vi "Event Structure Details.vi"() -> ()   [LabVIEW 2023]
panel:
  in  "State mashine Time out control":i32
  out "Numeric":i32
  in  "stop":bool
  in  "OK Button":bool
  out "time string":string
  out "Waveform Chart":dbl(graph)
  # "Виж разликата когато е -1 и > -1"
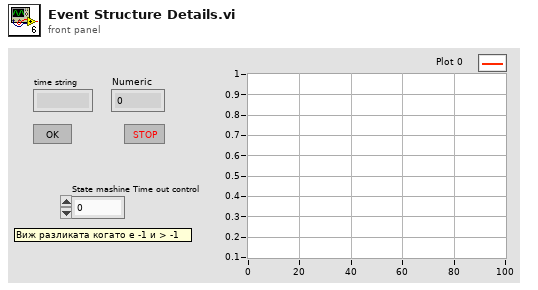
[diagram p1: front panel]
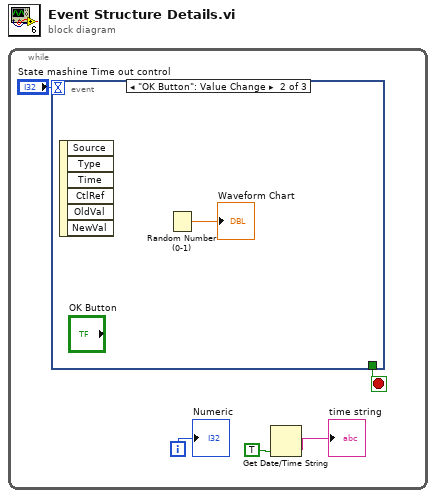
[diagram p0: block diagram]
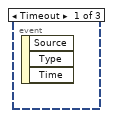
[diagram p2: hidden frame]
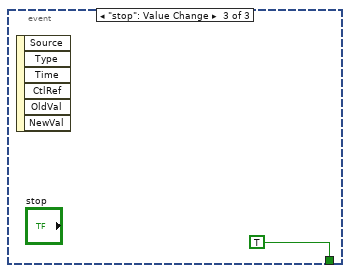
[diagram p3: hidden frame]
diagram:
  n1 = while {
    i -> [w3]
    stop <- w4 stop-if-true
    n2 = event shown="[1] \"OK Button\": Value Change" {
      selector: _ -> [_ _ _]
      dyn-events: _ -> [_ _ _]
      timeout: "State mashine Time out control" -> [_ _ _]
      tunnel: [_ _ TRUE] -> w4
      event Timeout {
        n3 = event-data() -> ()  [unwired: 1 in, 3 out]
      }
      event "OK Button": Value Change {
        n4 = event-data() -> ()  [unwired: 1 in, 6 out]
        n5 = Random Number (0-1)() -> (number: 0 to 1=→"Waveform Chart":dbl)
      }
      event "stop": Value Change {
        n6 = event-data() -> ()  [unwired: 1 in, 6 out]
      }
    }
    n7 = Get Date/Time String(want seconds? (F)=TRUE) -> (time string=→"time string":string)  [unwired: 2 in, 1 out]
    "Numeric" <- w3
  }
